vi "Read_Channels_CRGB.vi"(8 "error in (no error)":errorcluster, 11 "TCS3472 in":refnum<class "TCS3472.lvclass">) -> (0 "error out":errorcluster, 1 "Color":u32(colorbox), 2 "LightLevel":u8, 3 "TCS3472 out":refnum<class "TCS3472.lvclass">)   [LabVIEW 2020, in "TCS3472.lvclass"]
uses:
  TCS3472.lvclass
  TCS3472.lvclass/TCS3472.ctl
  Properties/Read LINX I2C.vi
  Properties/Write LINX I2C.vi
  LINX I2C/LINX I2C.lvclass
panel:
  out "REG_BLUE_L":u8 format="%02x"
  out "REG_GREEN_L":u8 format="%02x"
  out "REG_RED_L":u8 format="%02x"
  out "REG_CLEAR_L":u8 format="%02x"
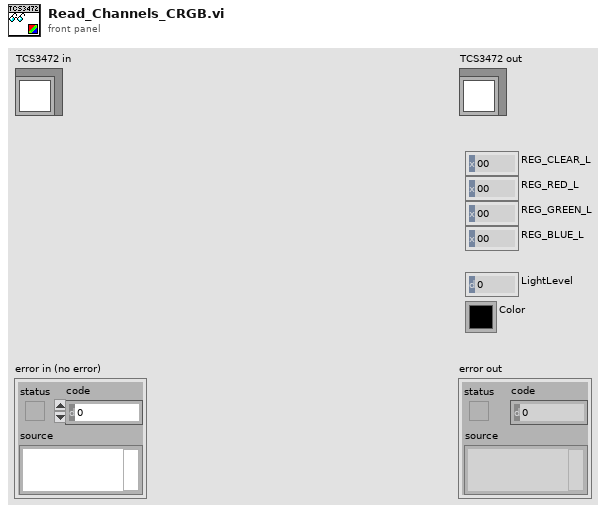
[diagram p1: front panel]
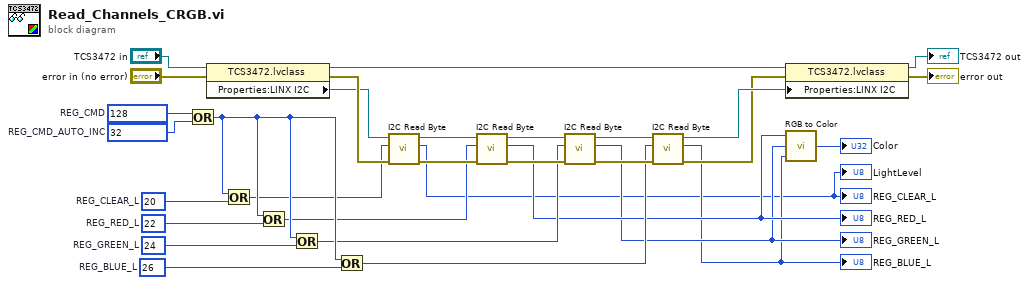
[diagram p0: block diagram]
diagram:
  w27 = u8 26  # REG_BLUE_L
  w26 = u8 24  # REG_GREEN_L
  w25 = u8 22  # REG_RED_L
  w28 = u8 20  # REG_CLEAR_L
  w29 = u8 32  # REG_CMD_AUTO_INC
  w30 = u8 128  # REG_CMD
  n1 = Or(x=w30, y=w29) -> (x .or. y?=w24:u8)
  n2 = property class="TCS3472.lvclass"(reference="TCS3472 in", error in="error in (no error)") -> (reference out=w20:refnum<class "TCS3472.lvclass">, error out=w23:errorcluster, "Properties:LINX I2C"=w18:refnum<class "LINX I2C.lvclass">)
  n3 = Or(x=w24, y=w28) -> (x .or. y?=w7:u8)
  n4 = Or(x=w24, y=w25) -> (x .or. y?=w9:u8)
  n5 = Or(x=w24, y=w26) -> (x .or. y?=w8:u8)
  n6 = Or(x=w24, y=w27) -> (x .or. y?=w6:u8)
  n7 = call-dynamic "I2C Read Byte.vi"("error in (no error)"=w23, "Register Address"=w7, "LINX I2C in"=w18) -> ("error out"=w14:errorcluster, "Byte Read"=→"REG_CLEAR_L" →"LightLevel":u8, "LINX I2C out"=w15:refnum<class "LINX I2C.lvclass">)  [unwired: 6 in]
  n8 = call-dynamic "I2C Read Byte.vi"("error in (no error)"=w14, "Register Address"=w9, "LINX I2C in"=w15) -> ("error out"=w12:errorcluster, "Byte Read"=w5:u8, "LINX I2C out"=w13:refnum<class "LINX I2C.lvclass">)  [unwired: 6 in]
  "REG_RED_L" <- w5
  n9 = call-dynamic "I2C Read Byte.vi"("error in (no error)"=w12, "Register Address"=w8, "LINX I2C in"=w13) -> ("error out"=w10:errorcluster, "Byte Read"=w4:u8, "LINX I2C out"=w11:refnum<class "LINX I2C.lvclass">)  [unwired: 6 in]
  "REG_GREEN_L" <- w4
  n10 = call-dynamic "I2C Read Byte.vi"("error in (no error)"=w10, "Register Address"=w6, "LINX I2C in"=w11) -> ("error out"=w16:errorcluster, "Byte Read"=w3:u8, "LINX I2C out"=w17:refnum<class "LINX I2C.lvclass">)  [unwired: 6 in]
  "REG_BLUE_L" <- w3
  n11 = property class="TCS3472.lvclass"(reference=w20, error in=w16, "Properties:LINX I2C"=w17) -> (reference out=→"TCS3472 out":refnum<class "TCS3472.lvclass">, error out=→"error out":errorcluster)
  n12 = call <vilib>:"RGB to Color.vi"("B"=w3, "G"=w4, "R"=w5) -> ("Color"=→"Color":u32)
